vi "2100_Test_Butterfly_SP3T.vi"(0 "Semiconductor Module Context":T6, 1 "current range":dbl=0.001 format="%#_6p", 2 "Master_Register_Data_Array_In":T1 {"Address" format="%.0x"}, 3 "current level":dbl=0.001 format="%#_13p", 5 "Script_Info":T4={"Script Name"="Butterfly", "All_Scripts"=[]}, 7 "Source Delay":dbl format="%#_6p", 9 "USID":T3 max=15, 11 "Error In":errorcluster, 12 "Instrument_Pins":T5={"SMU_Pins"=["RF1", "RF2", "RF3", "RF4"], "HSDIO_Pins"=["CLK", "SDA"]}, 13 "Thresholds(max R 1st)":dbl[](array[numeric])=[100000.0, 0.5], 14 "HV_Voltages":dbl[](array[numeric])) -> (6 "Master_Register_Data_Array_Out":T1 {"Address" format="%.0x"}, 15 "Error Out":errorcluster)   [LabVIEW 2013]
uses:
  Controls/USID.ctl
  <vilib>/NI_TestStand_SemiconductorModule/NI_TestStand_Semiconductor_Module.lvlibp/PinMap/General/SemiconductorModuleContext.ctl
  Controls/Master_Reg_Data_Array.ctl
  Controls/Reg_Address_Data.ctl
  <vilib>/NI_TestStand_SemiconductorModule/NI_TestStand_Semiconductor_Module.lvlibp/PinMap/General/Publish/PublishDataDoubleFunctionalTest.vi
  <vilib>/NI_TestStand_SemiconductorModule/NI_TestStand_Semiconductor_Module.lvlibp
panel:
  out "BF_Data to Log":dbl[](array[numeric])
  in  "Tab Control":enum32{"Test Info", "Instrument Settings"}(tab)
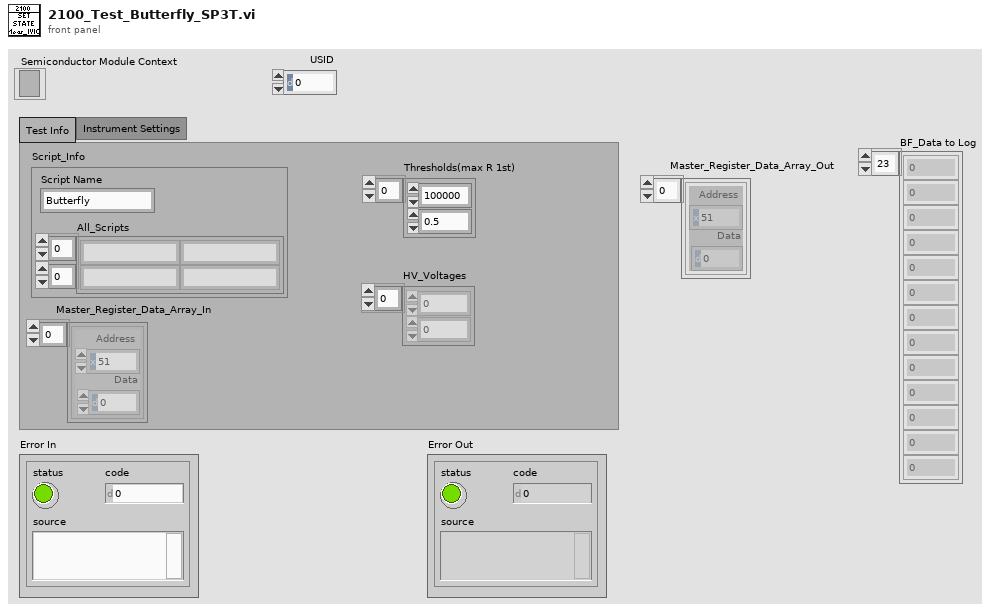
[diagram p1: front panel]
types:
  T1 = typedef "Master_Reg_Data_Array.ctl" = T2[]
  T2 = typedef "Reg_Address_Data.ctl" = cluster{"Address":u8, "Data":u8}
  T3 = typedef "USID.ctl" = u8
  T4 = cluster{"Script Name":string, "All_Scripts":string[][]}
  T5 = cluster{"SMU_Pins":string[], "HSDIO_Pins":string[]}
  T6 = typedef "NI_TestStand_Semiconductor_Module.lvlibp/SemiconductorModuleContext.ctl" = refnum<k7>
  T7 = typedef "Script Functions_Array.ctl" = enum16{"Reg_Write", "Bit_Write", "Delay", "Read", "Measure"}[]
  T8 = enum16{"Reg_Write", "Bit_Write", "Delay", "Read", "Measure"}
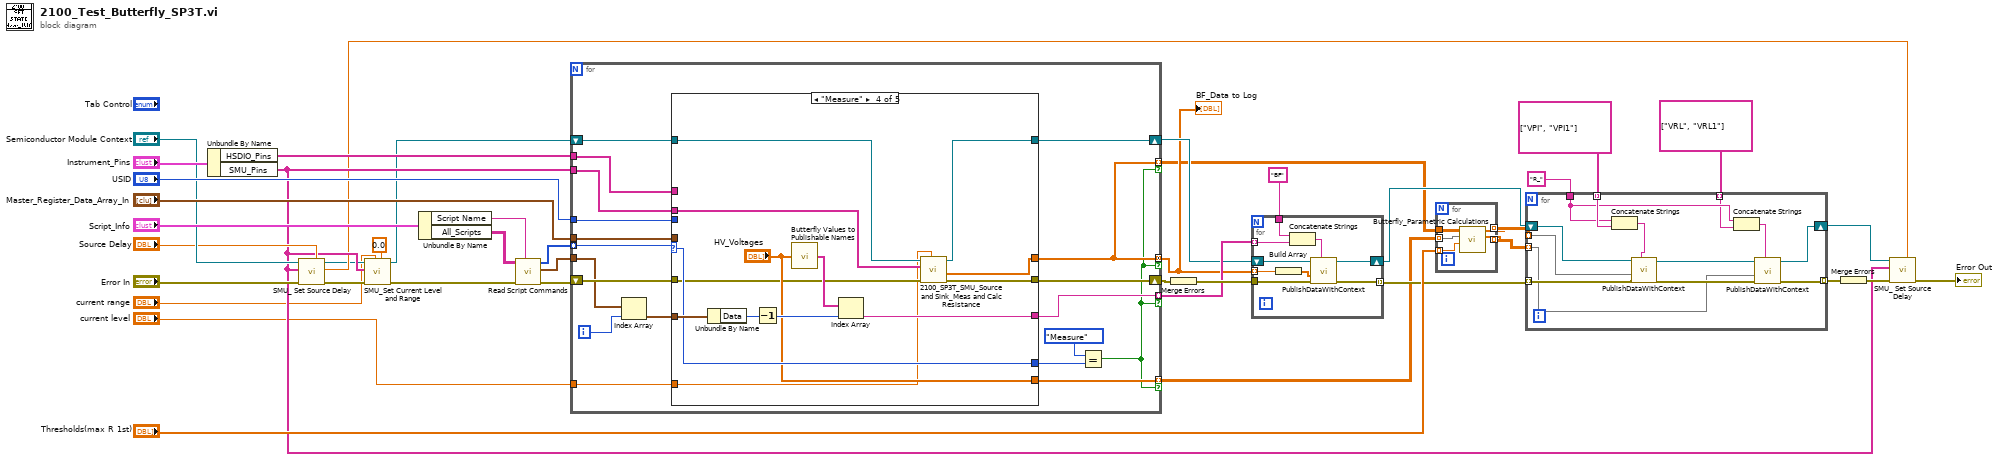
[diagram p0: block diagram]
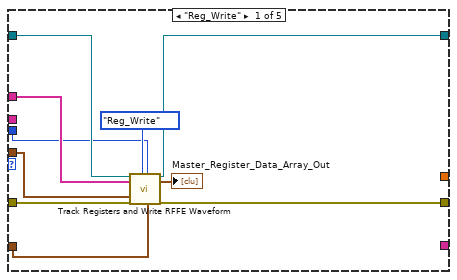
[diagram p2: hidden frame]
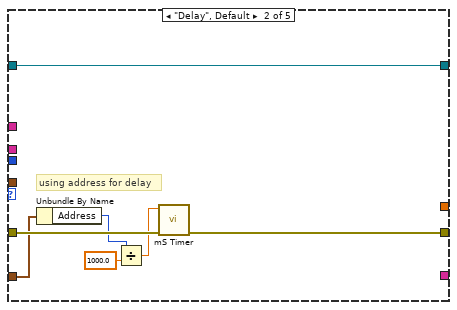
[diagram p3: hidden frame]
diagram:
  n1 = Unbundle By Name("Instrument_Pins") -> ("HSDIO_Pins"=w35:string[], "SMU_Pins"=w9:string[])
  n2 = call "SMU_ Set Source Delay.vi"("Source Delay"="Source Delay", "error in (no error)"="Error In", "Pins"=w9, "Semiconductor Module Context"="Semiconductor Module Context") -> ("error out"=w11:errorcluster, "Source Delay Readback"=w8:dbl, "Semiconductor Module Context Out"=w7:T6)  [unwired: 5 in]
  n3 = call "SMU_Set Current Level and Range.vi"("current level"=0.0, "current range"="current range", "error in (no error)"=w11, "Pins"=w9, "Semiconductor Module Context"=w7) -> ("error out"=w10:errorcluster, "Semiconductor Module Context Out"=w6:T6)  [unwired: 5 in]
  n4 = Unbundle By Name("Script_Info") -> ("Script Name"=w32:string, "All_Scripts"=w33:string[][])
  n5 = call "Read Script Commands.vi"("Test Name"=w32, "Error In"=w10, "All_Scripts"=w33) -> ("Error Out"=w39:errorcluster, "Script_Data"=w40:T2[], "Script_Functions"=w41:T7)  [unwired: 5 in, 1 out]
  n6 = for {
    tunnel: "USID" -> [w55]
    tunnel: w41 -> [w54] mode=indexing
    tunnel: w40 -> [w58]
    tunnel: w35 -> [w59]
    shift-right: [w52] -> w37
    shift-left: w39 -> [w61]
    tunnel: "Master_Register_Data_Array_In" -> [w56]
    tunnel: w9 -> [w51]
    shift-right: [w50] -> w15
    shift-left: w6 -> [w60]
    tunnel: [w44] -> w3 mode=concatenating if=w43
    tunnel: [w49] -> w16 mode=indexing if=w43
    tunnel: [w46] -> w12 mode=indexing if=w43
    tunnel: "current level" -> [w45]
    tunnel: [w44] -> w2 mode=indexing if=w43
    i -> [w53]
    n7 = Index Array(array=w58, index=w53) -> (element=w57:T2)
    n8 = case shown="\"Measure\"" w54 {
      selector: w54 -> [_ _ _ w89 _]
      tunnel: w57 -> [w66 w77 _ w94 _]
      tunnel: w61 -> [w71 w78 w80 w87 w96]
      tunnel: w55 -> [w63 _ _ _ _]
      tunnel: w60 -> [w69 w72 w79 w86 w95]
      tunnel: w59 -> [w68 _ _ _ _]
      tunnel: [w70 w76 w80 w84 w96] -> w52
      tunnel: w56 -> [w65 _ _ _ _]
      tunnel: w51 -> [_ _ _ w83 _]
      tunnel: [w62 w72 w79 w85 w95] -> w50
      tunnel: [_ _ _ w90 _] -> w49
      tunnel: [_ _ _ w89 _] -> w47
      tunnel: [_ _ _ "HV_Voltages" _] -> w46
      tunnel: [_ _ _ w82 _] -> w44
      tunnel: w45 -> [_ _ _ w81 _]
      frame "Reg_Write" {
        n9 = call "Track Registers and Write RFFE Waveform.vi"("Semiconductor Module Context"=w69, "Pins"=w68, "Master_Register_Data_Array_In"=w65, "Error In"=w71, "Script_Functions"=enum16{"Reg_Write", "Bit_Write"}."Reg_Write", "USID"=w63, "Reg_Address_Data"=w66) -> ("Semiconductor Module Context Out"=w62:T6, "Master_Register_Data_Array_Out"=→"Master_Register_Data_Array_Out":T1, "Error Out"=w70:errorcluster)  [unwired: 10 in]
      }
      frame "Delay", Default {
        # "using address for delay"
        n10 = Unbundle By Name(w77) -> ("Address"=w74:u8)
        n11 = Divide(x=w74, y=1000.0) -> (x/y=w73:dbl)
        n12 = call "mS Timer.vi"("Error In"=w78, "Delay(S)"=w73) -> ("Error Out"=w76:errorcluster)  [unwired: 9 in]
      }
      frame "Read" {
      }
      frame "Measure" {
        n13 = Unbundle By Name(w94) -> ("Data"=w93:u8)
        n14 = Decrement(x=w93) -> (x-1=w92:u8)
        n15 = call "Butterfly Values to Publishable Names.vi"("Butterfly Numbers"="HV_Voltages") -> ("Publishable Names"=w91:string[])
        n16 = Index Array(array=w91, index=w92) -> (element=w90:string)
        n17 = call "2100_SP3T_SMU_Source and Sink_Meas and Calc Resistance.vi"("Current  Level"=w81, "error in (no error)"=w87, "Pins"=w83, "Semiconductor Module Context"=w86) -> ("error Out"=w84:errorcluster, "Avg_Parallel_Calc"=w82:dbl[], "Semiconductor Module Context Out"=w85:T6)  [unwired: 4 in, 1 out]
      }
      frame "Bit_Write" {
      }
    }
    n18 = Equal?(x=T8."Measure" ("Enum"), y=w47) -> (x = y?=w43:bool)
  }
  "BF_Data to Log" <- w3
  n19 = Merge Errors(w37) -> (w18:errorcluster)
  n20 = for {
    tunnel: "BF" ("string") -> [w104]
    tunnel: w18 -> [w103]
    tunnel: [w102] -> w17 mode=indexing
    tunnel: w16 -> [w101] mode=indexing
    shift-right: [w99] -> w14
    shift-left: w15 -> [w100]
    tunnel: w3 -> [w98] mode=indexing
    n21 = Build Array(w98) -> (w97:dbl[])
    n22 = Concatenate Strings(w104, w101) -> (w105:string)
    n23 = call-poly <vilib>:"PublishDataWithContext.vi"("Published Data Id"=w105, "error in (no error)"=w103, "Data In"=w97, "Semiconductor Module Context"=w100) -> ("error out"=w102:errorcluster, "Semiconductor Module Context Out"=w99:T6)  [unwired: 6 in]
  }
  n24 = for {
    tunnel: [w110] -> w28 mode=indexing
    tunnel: [w109] -> w27 mode=indexing
    tunnel: "Thresholds(max R 1st)" -> [w108] mode=indexing
    tunnel: w12 -> [w107] mode=indexing
    tunnel: w2 -> [w106]
    n25 = call "Butterfly_Parametric Calculations.vi"("Threshold"=w108, "Voltage Array"=w107, "Result Array In"=w106) -> ("VRLs"=w109:dbl[], "VPIs"=w110:dbl[])  [unwired: 7 in]
  }
  n26 = for {
    tunnel: w17 -> [w123] mode=indexing
    tunnel: [w120] -> w26 mode=indexing
    tunnel: w28 -> [w118] mode=indexing
    tunnel: w27 -> [w117] mode=indexing
    tunnel: string[] ["VPI", "VPI1"] -> [w115] mode=indexing
    tunnel: string[] ["VRL", "VRL1"] -> [w111] mode=indexing
    shift-right: [w116] -> w20
    shift-left: w14 -> [w122]
    tunnel: "R_" ("string") -> [w112]
    n27 = Concatenate Strings(w112, w115) -> (w114:string)
    n28 = call-poly <vilib>:"PublishDataWithContext.vi"("Published Data Id"=w114, "error in (no error)"=w123, "Data In"=w118, "Semiconductor Module Context"=w122) -> ("error out"=w121:errorcluster, "Semiconductor Module Context Out"=w119:T6)  [unwired: 6 in]
    n29 = Concatenate Strings(w112, w111) -> (w113:string)
    n30 = call-poly <vilib>:"PublishDataWithContext.vi"("Published Data Id"=w113, "error in (no error)"=w121, "Data In"=w117, "Semiconductor Module Context"=w119) -> ("error out"=w120:errorcluster, "Semiconductor Module Context Out"=w116:T6)  [unwired: 6 in]
  }
  n31 = Merge Errors(w26) -> (w22:errorcluster)
  n32 = call "SMU_ Set Source Delay.vi"("Source Delay"=w8, "error in (no error)"=w22, "Pins"=w9, "Semiconductor Module Context"=w20) -> ("error out"=→"Error Out":errorcluster)  [unwired: 5 in, 2 out]
